vi "SRV_Sensor PARSE_##ib.vi"(0 "Return Data":string) -> (3 "Constant Command":string, 10 "Value":u8)   [LabVIEW 2009]
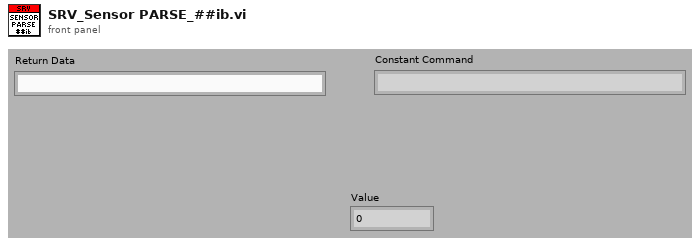
[diagram p1: front panel]
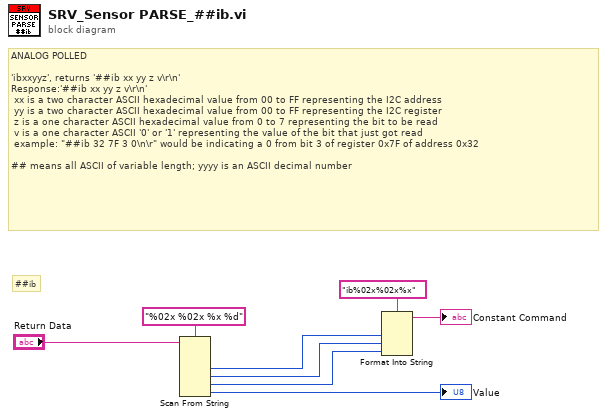
[diagram p0: block diagram]
diagram:
  # "##ib"
  # "ANALOG POLLED\n\n'ibxxyyz', returns '##ib xx yy z v\\r\\n'\nResponse:'##ib xx yy z v\\r\\n'\n xx is a two character ASCII hexadecimal value from 00 to FF representing the I2C address\n yy is a two character ASCII hexadecimal value from 00 to FF representing the I2C register\n z is a one character ASCII hexadecimal value from 0 to 7 representing the bit to be read\n v is a one character ASCII '0' or '1' representing the value of the bit that just got read\n example: \"##ib 32 7F 3 0\\n\\r\" would be indicating a 0 from bit 3 of register 0x7F of address 0x32\n\n## means all ASCII of variable length; yyyy is an ASCII decimal number"
  n1 = Scan From String(format string="%02x %02x %x %d", input string="Return Data") -> (output 1=w3:i32, output 2=w2:i32, output 3=w1:i32, output 4=→"Value":u8)  [unwired: 6 in, 3 out]
  n2 = Format Into String(format string="ib%02x%02x%x", w3, w2, w1) -> (resulting string=→"Constant Command":string)  [unwired: 2 in, 1 out]
